vi "NumIntegrate_Func_Ct.vi"(11 "Index":i32) -> (3 "Ct":dbl)   [LabVIEW 2019, in "Trajectory_Library.lvlib"]
doc: "Creates a new LINEAR SYSTEM data cluster with the specified values. \n\n\nInputs: \n - XXX -- XXX.\n\nOutputs:\n - XXX -- XXX."
uses:
  Trajectory_Library.lvlib
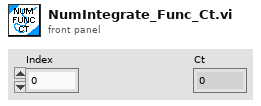
[diagram p1: front panel]
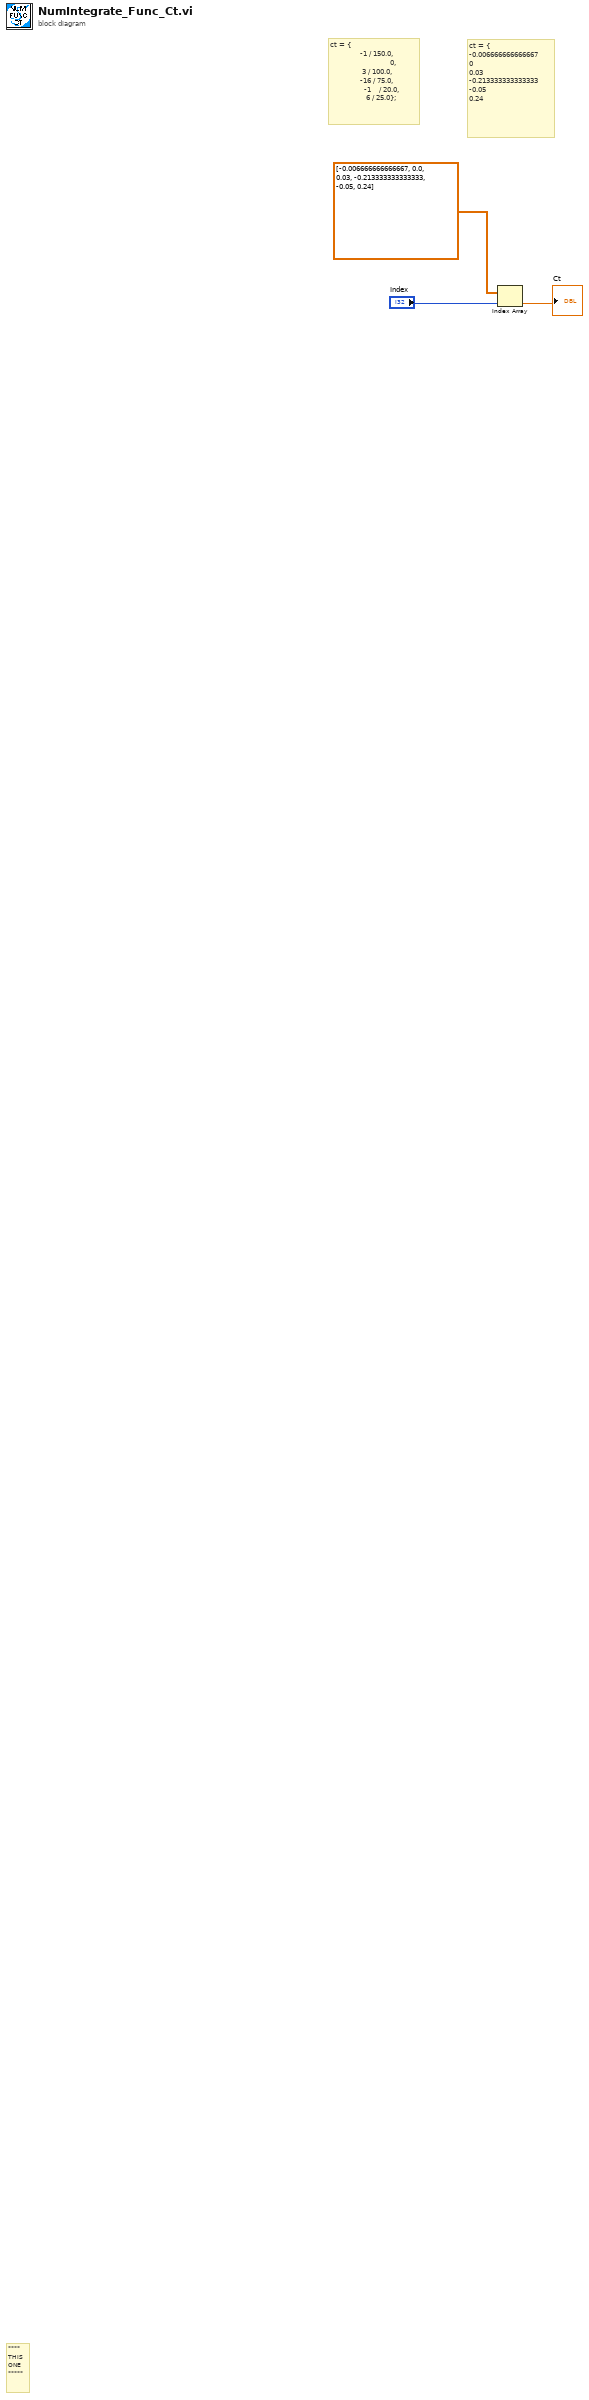
[diagram p0: block diagram]
diagram:
  # "ct = {\n-0.006666666666667\n0\n0.03\n-0.213333333333333\n-0.05\n0.24"
  # "ct = {\n               -1 / 150.0, \n                              0, \n                3 / 100.0, \n               -16 / 75.0, \n                 -1    / 20.0, \n                  6 / 25.0};"
  # "****\nTHIS\nONE\n*****"
  n1 = Index Array(array=dbl[] [-0.006666666666667, 0.0, 0.03, -0.213333333333333, -0.05, 0.24], index="Index") -> (element=→"Ct":dbl)
